vi "HB_LogLineSD.vi"(8 "error in (no error)":errorcluster, 10 "Log string":string, 11 "HBDevRef":T1) -> (0 "error out":errorcluster, 3 "HBDevRef":T1)   [LabVIEW 2016]
doc: "Logs the specified string to the currently opened file on the SD card. If no file has been opened, the specified string will not be logged. The length of the string must be less than 246 characters or else no data will be logged."
uses:
  <vilib>/Rock Robotics/WPI/SerialPort/WPI_SerialPortRef.ctl
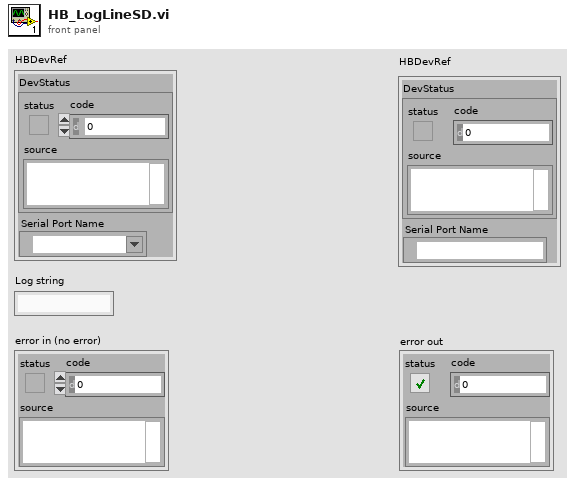
[diagram p1: front panel]
types:
  T1 = typedef "WPI_SerialPortRef.ctl" = cluster{"DevStatus":errorcluster, "Serial Port Name":refnum<visa-resource-name>}
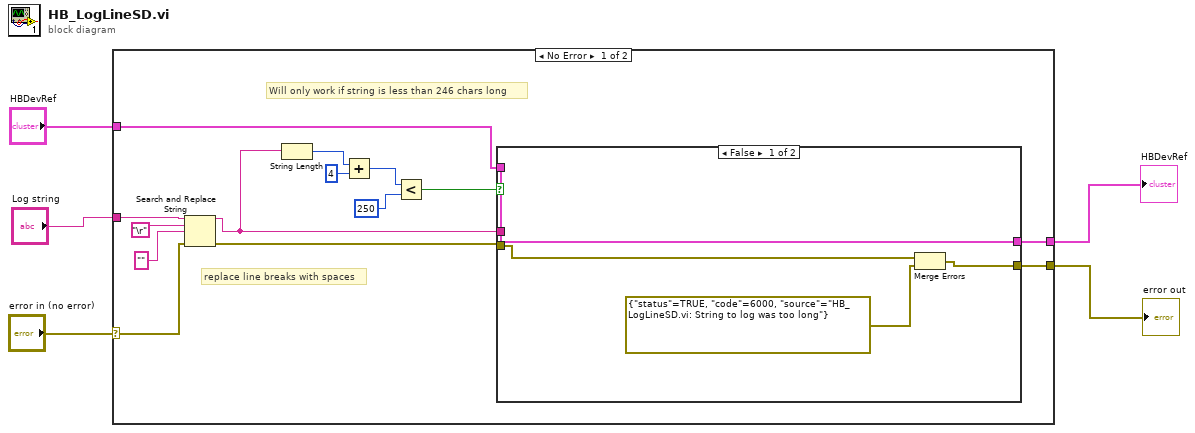
[diagram p0: block diagram]
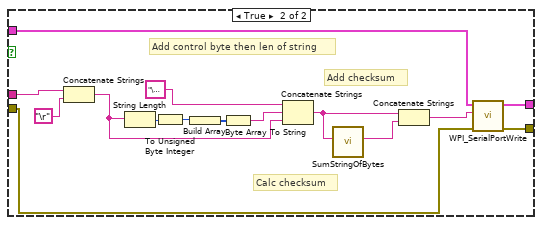
[diagram p2: hidden frame]
diagram:
  n1 = case shown="No Error" "error in (no error)" {
    selector: "error in (no error)" -> [w6 w40]
    tunnel: "Log string" -> [w18 _]
    tunnel: "HBDevRef" -> [w9 w39]
    tunnel: [w8 w39] -> w3
    tunnel: [w7 w40] -> w2
    frame No Error {
      # "Will only work if string is less than 246 chars long"
      # "replace line breaks with spaces"
      n2 = Search and Replace String(input string=w18, search string="\r", replace string="" ("replace string (\"\")"), error in=w6) -> (result string=w12:string, error out=w11:errorcluster)  [unwired: 4 in, 2 out]
      n3 = String Length(string=w12) -> (length=w14:i32)
      n4 = Add(x=w14, y=4) -> (x+y=w16:i32)
      n5 = Less?(x=w16, y=250) -> (x < y?=w13:bool)
      n6 = case shown="False" w13 {
        tunnel: w12 -> [_ w25]
        tunnel: w11 -> [w21 w24]
        tunnel: [w20 w28] -> w8
        tunnel: [w22 w27] -> w7
        tunnel: w9 -> [w20 w26]
        frame False {
          n7 = Merge Errors(w21, errorcluster {"status"=TRUE, "code"=6000, "source"="HB_LogLineSD.vi: String to log was too long"} ("error out")) -> (w22:errorcluster)
        }
        frame True {
          # "Add checksum"
          # "Add control byte then len of string"
          # "Calc checksum"
          n8 = Concatenate Strings(w25, "\r") -> (w31:string)
          n9 = String Length(string=w31) -> (length=w33:i32)
          n10 = To Unsigned Byte Integer(number=w33) -> (unsigned 8bit integer=w32:u8)
          n11 = Build Array(w32) -> (w38:u8[])
          n12 = Byte Array To String(unsigned byte array=w38) -> (string=w37:string)
          n13 = Concatenate Strings("\u0001", w37, w31) -> (w34:string)
          n14 = call "SumStringOfBytes.vi"("String Of Bytes"=w34) -> ("SumAsString"=w35:string)  [unwired: 10 in]
          n15 = Concatenate Strings(w34, w35) -> (w29:string)
          n16 = call <vilib>:"WPI_SerialPortWrite.vi"("error in (no error)"=w24, "Buffer"=w29, "SerialPortRef"=w26) -> ("error out"=w27:errorcluster, "SerialPortRef"=w28:T1)  [unwired: 6 in, 1 out]
        }
      }
    }
    frame Error {
    }
  }
  "HBDevRef" <- w3
  "error out" <- w2
